vi "DAQ_Grab.vi"(6 "Input":u16(ring) items=["Hammer (force)", "Self-tap"], 8 "error In":errorcluster, 9 "Threshold":dbl, 10 "Pre-trigger (s)":dbl=0.01 format="%#_13g", 11 "DAQ Prams":T3={"task in"="", "Num Pts"=0, "timeout"=0.0, "FIFO"=0, "Double Bounce"=1.0, "Sensitivity (V/X)"=[]} {"Double Bounce" format="%#.2g"}) -> (0 "error out":errorcluster, 1 "Buffer":waveform(dbl)[](array[waveform]), 2 "Full":bool, 3 "DAQ Prams":T3={"task in"="", "Num Pts"=0, "timeout"=0.0, "FIFO"=0, "Double Bounce"=1.0, "Sensitivity (V/X)"=[]} {"Double Bounce" format="%#.2g"}, 4 "Start Task":T2(ring), 5 "Tap":T1)   [LabVIEW 2022 SP3]
uses:
  <vilib>/Waveform/WDTOps.llb/WDT Append Waveforms DBL.vi
  <extravilib>/ChannelInstances/Lossy Stream-a[.](wfm(dbl)).lvlib
  Mic_Global.vi
  <vilib>/DAQmx/read.llb/DAQmx Read (Analog 1D Wfm NChan NSamp).vi
  <extravilib>/ChannelInstances/Lossy Stream-a[.](wfm(dbl))/)Channel.ctl
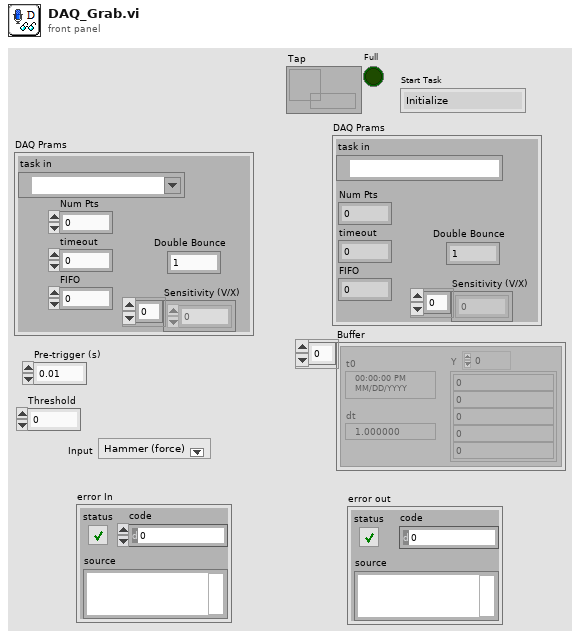
[diagram p1: front panel]
types:
  T1 = typedef "Lossy Stream-a[.](wfm(dbl)).lvlib/)Channel.ctl" = refnum<queue>
  T2 = enum16{"Initialize", "Free run", "One Shot - waiting", "One Shot - triggered", "Wait", "Close"}
  T3 = cluster{"task in":refnum<k21>, "Num Pts":i32, "timeout":dbl, "FIFO":i32, "Double Bounce":dbl, "Sensitivity (V/X)":dbl[]}
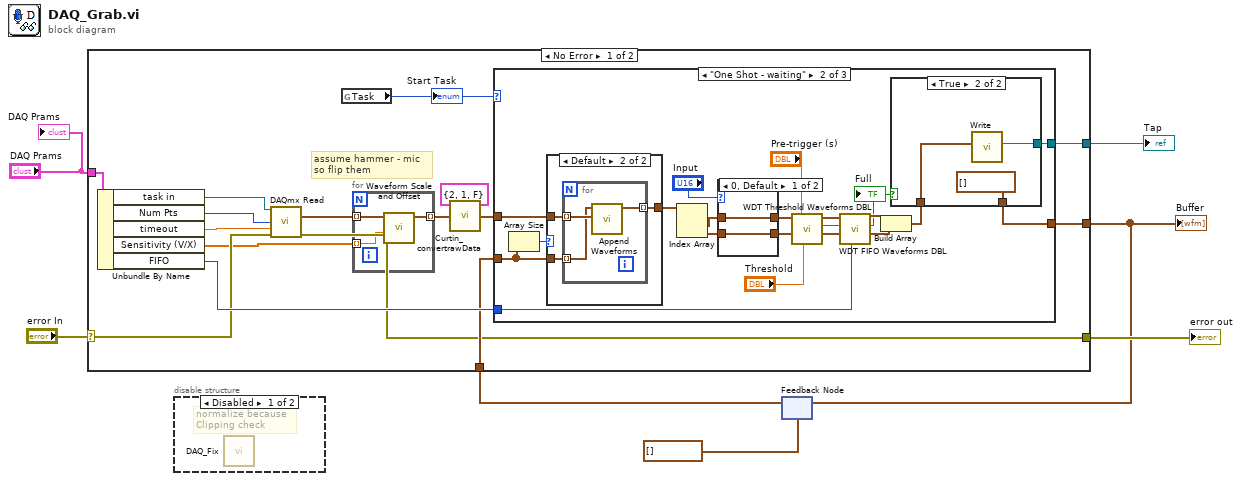
[diagram p0: block diagram]
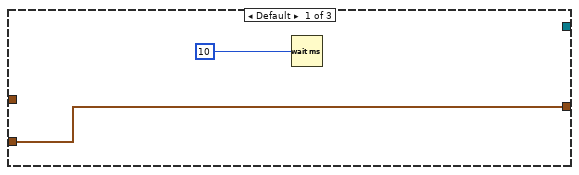
[diagram p3: hidden frame]
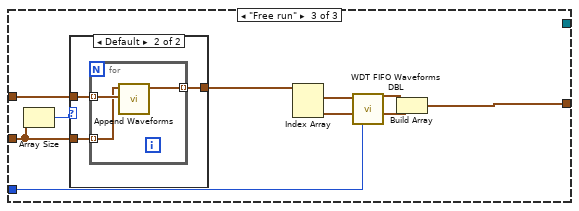
[diagram p7: hidden frame]
diagram:
  n1 = disable-structure shown="Disabled" {
    frame Disabled {
      # "normalize because\nClipping check"
      n2 = call "DAQ_Fix.vi"() -> ()  [unwired: 11 in, 1 out]
    }
    frame Enabled {
    }
  }
  n3 = feedback #1(waveform(dbl)[] []) -> (w5:waveform(dbl)[])
  n4 = case shown="No Error" "error In" {
    selector: "error In" -> [w9 w81]
    tunnel: "DAQ Prams" -> [w23 _]
    tunnel: [w16 w81] -> w7
    tunnel: [w21 w82] -> w6
    tunnel: w5 -> [w20 w82]
    tunnel: [w17 _] -> w2
    frame No Error {
      # "assume hammer - mic\nso flip them"
      n5 = Unbundle By Name(w23) -> ("task in"=w13:refnum<k21>, "Num Pts"=w15:i32, "timeout"=w14:dbl, "Sensitivity (V/X)"=w8:dbl[], "FIFO"=w22:i32)
      n6 = call-poly <vilib>:"DAQmx Read.vi"("task/channels in"=w13, "number of samples per channel"=w15, "timeout"=w14, "error in"=w9) -> ("data"=w11:waveform(dbl)[], "error out"=w16:errorcluster)  [unwired: 9 in, 1 out]
      n7 = global read "Mic_Global.vi" "Task"() -> (w19:T2)
      "Start Task" <- w19
      n8 = for {
        tunnel: w11 -> [w26] mode=indexing
        tunnel: [w25] -> w10 mode=indexing
        tunnel: w8 -> [w24] mode=indexing
        n9 = call <vilib>:"Waveform Scale and Offset.vi"("scale"=w24, "waveform in"=w26) -> ("waveform out"=w25:waveform(dbl))  [unwired: 8 in, 1 out]
      }
      n10 = call "Curtin_convertrawData.vi"("incoming data"=w10, "Ports"=cluster{"Ch_1":u8, "Ch_2":u8, bool} {"Ch_1"=2, "Ch_2"=1, FALSE}) -> ("Ordered"=w12:waveform(dbl)[])
      n11 = case shown="\"One Shot - waiting\"" w19 {
        tunnel: w12 -> [_ w49 w73]
        tunnel: w20 -> [w28 w41 w66]
        tunnel: [w28 w34 w64] -> w21
        tunnel: w22 -> [_ w42 w69]
        tunnel: [_ w35 _] -> w17
        frame Default {
          n12 = Wait (ms)(milliseconds to wait=u32 10) -> ()  [unwired: 1 out]
        }
        frame "One Shot - waiting" {
          n13 = Array Size(array=w41) -> (size(s)=w40:i32)
          n14 = case shown="Default" w40 {
            tunnel: w49 -> [w57 w60]
            tunnel: w41 -> [_ w59]
            tunnel: [w57 w58] -> w43
            frame 0 {
            }
            frame Default {
              n15 = for {
                tunnel: w60 -> [w63] mode=indexing
                tunnel: [w62] -> w58 mode=indexing
                tunnel: w59 -> [w61] mode=indexing
                n16 = call-poly <vilib>:"Append Waveforms.vi"("waveform B"=w63, "waveform A"=w61) -> ("waveform out"=w62:waveform(dbl))  [unwired: 8 in, 1 out]
              }
            }
          }
          n17 = Index Array(array=w43) -> (element #1=w29:waveform(dbl), element #2=w31:waveform(dbl))  [unwired: 2 in]
          n18 = case shown="0, Default" "Input" {
            tunnel: [w51 w52] -> w32
            tunnel: w31 -> [w50 _]
            tunnel: [w50 w52] -> w30
            tunnel: w29 -> [w51 w52]
            frame 0, Default {
            }
            frame 1 {
            }
          }
          n19 = call "WDT Threshold Waveforms DBL.vi"("A Threshold"="Threshold", "Pre-trigger (s)"="Pre-trigger (s)", "Hammer"=w30, "Mic"=w32) -> ("Hammer out"=w48:waveform(dbl), "Triggered?"=w44:bool, "Mic out"=w47:waveform(dbl))  [unwired: 4 in, 1 out]
          n20 = call "WDT FIFO Waveforms DBL.vi"("FIFO"=w42, "Hammer"=w48, "Triggered?"=w44, "Mic"=w47) -> ("Hammer out"=w46:waveform(dbl), "Full"=w39:bool, "Mic out"=w45:waveform(dbl))  [unwired: 4 in, 1 out]
          "Full" <- w39
          n21 = Build Array(w45, w46) -> (w36:waveform(dbl)[])
          n22 = case shown="True" w39 {
            tunnel: w36 -> [w53 w54]
            tunnel: [_ w56] -> w35
            tunnel: [w53 waveform(dbl)[] []] -> w34
            frame False {
            }
            frame True {
              n23 = call <extravilib>:"Write.vi"("element"=w54) -> ("channel"=w56:T1)  [unwired: 8 in, 2 out]
            }
          }
        }
        frame "Free run" {
          n24 = Array Size(array=w66) -> (size(s)=w65:i32)
          n25 = case shown="Default" w65 {
            tunnel: w73 -> [w74 w77]
            tunnel: w66 -> [_ w76]
            tunnel: [w74 w75] -> w70
            frame 0 {
            }
            frame Default {
              n26 = for {
                tunnel: w77 -> [w80] mode=indexing
                tunnel: [w79] -> w75 mode=indexing
                tunnel: w76 -> [w78] mode=indexing
                n27 = call-poly <vilib>:"Append Waveforms.vi"("waveform B"=w80, "waveform A"=w78) -> ("waveform out"=w79:waveform(dbl))  [unwired: 8 in, 1 out]
              }
            }
          }
          n28 = Index Array(array=w70) -> (element #1=w68:waveform(dbl), element #2=w67:waveform(dbl))  [unwired: 2 in]
          n29 = call "WDT FIFO Waveforms DBL.vi"("FIFO"=w69, "Hammer"=w67, "Mic"=w68) -> ("Hammer out"=w72:waveform(dbl), "Mic out"=w71:waveform(dbl))  [unwired: 5 in, 2 out]
          n30 = Build Array(w71, w72) -> (w64:waveform(dbl)[])
        }
      }
    }
    frame Error {
    }
  }
  "Buffer" <- w6
  "error out" <- w7
  "Tap" <- w2
  n31 = feedback-in #1(w6) -> ()
  "DAQ Prams" <- "DAQ Prams"
